vi "ShiftAlongX.vi"(0 "Data":cluster{cluster{dbl, dbl}[]}[](array[cluster]), 3 "X shift":dbl) -> (14 "Data":cluster{cluster{dbl, dbl}[]}[](array[cluster]))   [LabVIEW 2018]
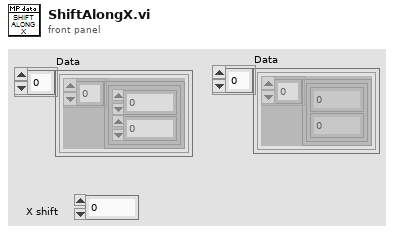
[diagram p1: front panel]
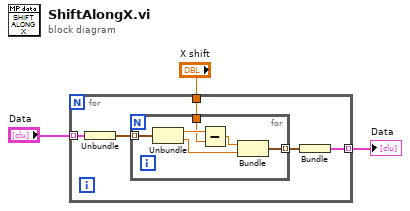
[diagram p0: block diagram]
diagram:
  n1 = for {
    tunnel: "Data" -> [w8] mode=indexing
    tunnel: "X shift" -> [w6]
    tunnel: [w4] -> w1 mode=indexing
    n2 = Unbundle(w8) -> (w7:cluster{dbl, dbl}[])
    n3 = for {
      tunnel: w7 -> [w14] mode=indexing
      tunnel: w6 -> [w12]
      tunnel: [w9] -> w5 mode=indexing
      n4 = Unbundle(w14) -> (w13:dbl, w10:dbl)
      n5 = Subtract(x=w13, y=w12) -> (x-y=w11:dbl)
      n6 = Bundle(w11, w10) -> (w9:cluster{dbl, dbl})  [unwired: 1 in]
    }
    n7 = Bundle(w5) -> (w4:cluster{cluster{dbl, dbl}[]})  [unwired: 1 in]
  }
  "Data" <- w1
